vi "put_cushion.vi"(8 "error in (no error)":errorcluster, 11 "IChair.lvclass":refnum<class "IChair.lvclass">) -> (0 "error out":errorcluster, 1 "result":string, 3 "IChair.lvclass":refnum<class "IChair.lvclass">)   [LabVIEW 2021, in "IChair.lvclass"]
uses:
  IChair.lvclass
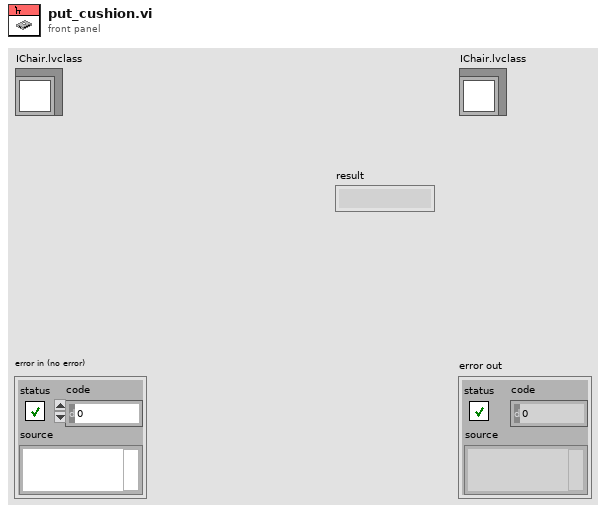
[diagram p1: front panel]
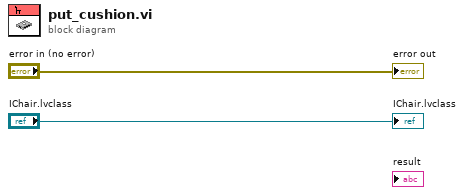
[diagram p0: block diagram]
diagram:
  "error out" <- "error in (no error)"
  "IChair.lvclass" <- "IChair.lvclass"
